vi "Get Case Structure Frame (by Name).vi"(8 "error in (no error)":errorcluster, 10 "element":string, 11 "CaseStructure in":refnum<vi>) -> (0 "error out":errorcluster, 1 "Found?":bool, 2 "Frame ref out":refnum<vi>, 3 "CaseStructure out":refnum<vi>)   [LabVIEW 2019, in "gRPC Template Creation Utility.lvlib"]
uses:
  gRPC Template Creation Utility.lvlib
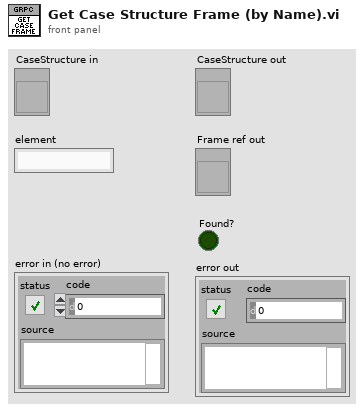
[diagram p1: front panel]
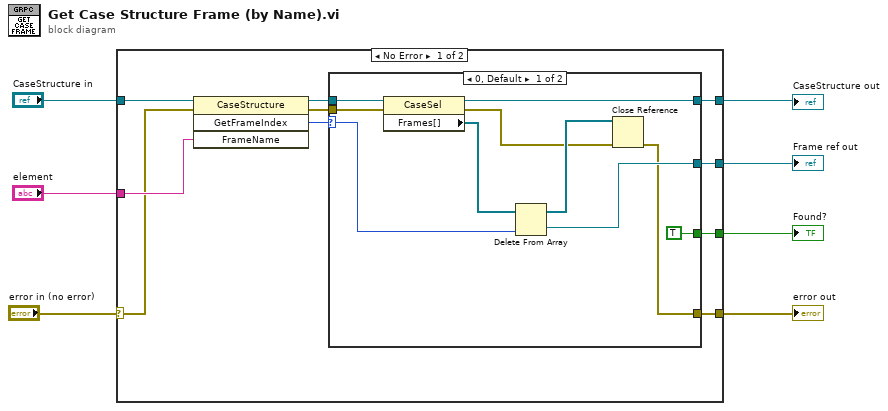
[diagram p0: block diagram]
diagram:
  n1 = case shown="No Error" "error in (no error)" {
    selector: "error in (no error)" -> [w10 w31]
    tunnel: "CaseStructure in" -> [w17 w30]
    tunnel: [w16 _] -> w6
    tunnel: [w15 w30] -> w5
    tunnel: [w14 w31] -> w4
    tunnel: "element" -> [w12 _]
    tunnel: [w8 _] -> w1
    frame No Error {
      n2 = invoke class="CaseStructure" method="GetFrameIndex"(reference=w17, error in=w10, "FrameName"=w12) -> (reference out=w13:refnum<vi>, error out=w11:errorcluster, "GetFrameIndex"=w9:i32)  [unwired: 1 in, 1 out]
      n3 = case shown="0, Default" w9 {
        selector: w9 -> [w19 _]
        tunnel: [w27 _] -> w16
        tunnel: [w26 w29] -> w15
        tunnel: [w25 w28] -> w14
        tunnel: w13 -> [w22 w29]
        tunnel: w11 -> [w21 w28]
        tunnel: [TRUE _] -> w8
        frame 0, Default {
          n4 = property class="CaseSel"(reference=w22, error in=w21) -> (reference out=w26:refnum<vi>, error out=w20:errorcluster, "Frames[]"=w23:refnum<vi>[])
          n5 = Delete From Array(array=w23, index=w19) -> (deleted portion=w27:refnum<vi>, array with subset deleted=w24:refnum<vi>[])  [unwired: 1 in]
          n6 = Close Reference(reference=w24, error in (no error)=w20) -> (error out=w25:errorcluster)
        }
        frame -1 {
        }
      }
    }
    frame Error {
    }
  }
  "Frame ref out" <- w6
  "CaseStructure out" <- w5
  "error out" <- w4
  "Found?" <- w1
